vi "tm_getvaluetext_40.vi"(2 "Value in":dbl, 7 "Reconfigure (F)":bool, 8 "error in (no error)":errorcluster, 10 "Parameter":u32(ring)=4215968 items=["SENSOR MODE"=4212128, "READOUT SPEED"=4211872, "READOUT DIRECTION"=4211904, "TRIGGER GLOBAL EXPOSURE"=2049680, "TRIGGER DELAY"=1066480, "INTERNAL TRIGGER HANDLING"=1066496, "SYNC READOUT SYSTEM BLANK"=1066528, "SENSOR TEMPERATURE"=2115232, "SENSOR COOLER STATUS"=2115280, "EXPOSURE TIME"=2049184, "DEFECT CORRECT MODE"=4670368, "BINNING"=4215968, "INTERNAL LINE SPEED"=4226000, "INTERNAL LINE INTERVAL"=4226016, "NUMBER OF OUTPUT TRIGGER CONNECTOR"=1852320, "OUTPUT TRIGGER SOURCE[0]"=1852576, "OUTPUT TRIGGER SOURCE[1]"=1852832, "OUTPUT TRIGGER SOURCE[2]"=1853088, "OUTPUT TRIGGER POLARITY[0]"=1852592, "OUTPUT TRIGGER POLARITY[1]"=1852848, "OUTPUT TRIGGER POLARITY[2]"=1853104, "OUTPUT TRIGGER ACTIVE[0]"=1852608, "OUTPUT TRIGGER ACTIVE[1]"=1852864, "OUTPUT TRIGGER ACTIVE[2]"=1853120, "OUTPUT TRIGGER DELAY[0]"=1852624, "OUTPUT TRIGGER DELAY[1]"=1852880, "OUTPUT TRIGGER DELAY[2]"=1853136, "OUTPUT TRIGGER PERIOD[0]"=1852640, "OUTPUT TRIGGER PERIOD[1]"=1852896, "OUTPUT TRIGGER PERIOD[2]"=1853152, "OUTPUT TRIGGER KIND[0]"=1852656, "OUTPUT TRIGGER KIND[1]"=1852912, "OUTPUT TRIGGER KIND[2]"=1853168, "OUTPUT TRIGGER BASE SENSOR[0]"=1852672, "OUTPUT TRIGGER BASE SENSOR[1]"=1852928, "OUTPUT TRIGGER BASE SENSOR[2]"=1853184, "OUTPUT TRIGGER PRE HSYNC COUNT"=1852704], 11 "Handle in":u32) -> (0 "error out":errorcluster, 3 "Handle out":u32)   [LabVIEW 2023]
uses:
  tmcamcon.dll
panel:
  out "Text Value":string
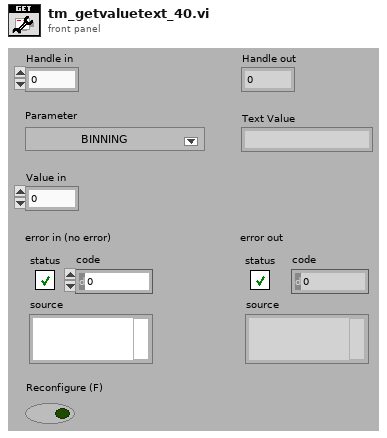
[diagram p1: front panel]
types:
  T1 = cluster{"Property Name":string, "Property ID":i32}[]
  T2 = cluster{"Property Name":string, "Property ID":i32}
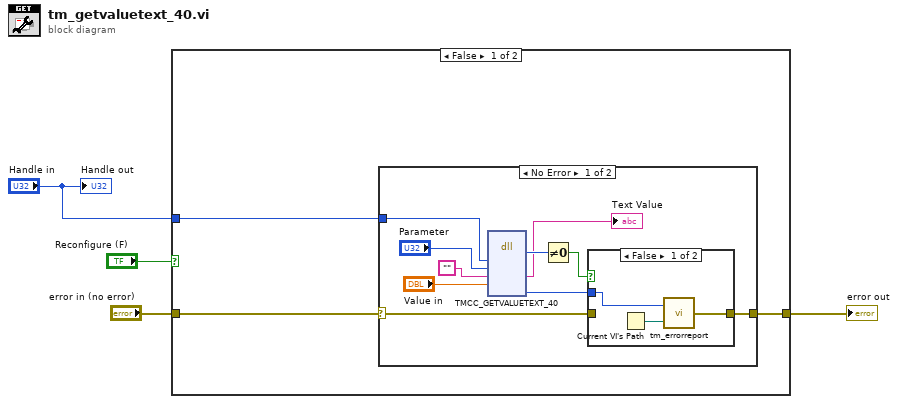
[diagram p0: block diagram]
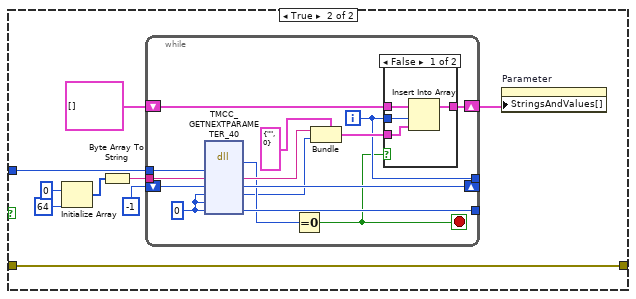
[diagram p4: hidden frame]
diagram:
  n1 = case shown="False" "Reconfigure (F)" {
    tunnel: "error in (no error)" -> [w6 w31]
    tunnel: [w7 w31] -> w3
    tunnel: "Handle in" -> [w5 w23]
    frame False {
      n2 = case shown="No Error" w6 {
        selector: w6 -> [w15 w22]
        tunnel: [w12 w22] -> w7
        tunnel: w5 -> [w16 _]
        frame No Error {
          n3 = dll-call lib="tmcamcon.dll" fn="TMCC_GETVALUETEXT_40"("handle"=w16, "parameter"="Parameter", "text"="", "value"="Value in") -> ("return type"=w17:u32, "text"=→"Text Value":string, "Erval"=w14:i32)  [unwired: 7 in, 2 out]
          n4 = Not Equal To 0?(x=w17) -> (x != 0?=w13:bool)
          n5 = case shown="False" w13 {
            tunnel: w15 -> [_ w21]
            tunnel: [w19 w21] -> w12
            tunnel: w14 -> [w18 _]
            frame False {
              n6 = Current VI's Path() -> (path=w20:path)
              n7 = call "tm_errorreport.vi"("Source"=w20, "Error"=w18) -> ("error out"=w19:errorcluster)
            }
            frame True {
            }
          }
        }
        frame Error {
        }
      }
    }
    frame True {
      n8 = Initialize Array(u8 0 ("element"), 64 ("dimension size")) -> (w26:u8[])
      n9 = Byte Array To String(unsigned byte array=w26) -> (string=w29:string)
      n10 = while {
        shift-right: [w45] -> w24
        shift-left: T1 [] ("Array") -> [w46]
        tunnel: [w41] -> _
        tunnel: [w39] -> _
        tunnel: w29 -> [w38]
        tunnel: w23 -> [w37]
        shift-right: [w40] -> _
        shift-left: -1 ("func_num") -> [w42]
        i -> [w39]
        stop <- w35 stop-if-true
        w32 = 0 ("option")
        n11 = dll-call lib="tmcamcon.dll" fn="TMCC_GETNEXTPARAMETER_40"("HDCAM"=w37, "name"=w38, "func_num"=w42, "func_id"=w32, "option"=w32, "Erval"=w32) -> ("return type"=w34:u32, "name"=w43:string, "func_num"=w40:i32, "func_id"=w33:i32, "Erval"=w41:i32)  [unwired: 5 in, 2 out]
        n12 = Equal To 0?(x=w34) -> (x = 0?=w35:bool)
        n13 = Bundle(cluster=T2 {"Property Name"="", "Property ID"=0} ("new element/subarray"), "Property Name"=w43, "Property ID"=w33) -> (w44:T2)
        n14 = case shown="False" w35 {
          tunnel: w46 -> [w50 w51]
          tunnel: [w49 w51] -> w45
          tunnel: w39 -> [w48 _]
          tunnel: w44 -> [w47 _]
          frame False {
            n15 = Insert Into Array(array=w50, index=w48, new element=w47) -> (w49:T1)
          }
          frame True {
          }
        }
      }
      n16 = property on="Parameter" class="Ring (strict)"("StringsAndValues[]"=w24) -> ()  [unwired: 2 in, 2 out]
    }
  }
  "error out" <- w3
  "Handle out" <- "Handle in"
